vi "Global_FPGA.vi"() -> ()   [LabVIEW 2015]
panel:
  out "QPD":T1
  out "FPGA ready":bool
  out "FPGA done":bool
  out "FPGA start":bool
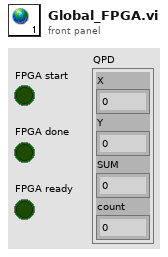
[diagram p1: front panel]
types:
  T1 = cluster{"X":sgl, "Y":sgl, "SUM":sgl, "count":u32}
diagram:
